vi "WS1050 VPI CP Sweep Cmd.vi"(8 "error in (no error)":errorcluster, 11 "x":dbl=23.0) -> (0 "error out":errorcluster, 2 "Bi_Voltage Out":string[](array[string]), 3 "Bi_Cmd Out":string[](array[string]), 4 "CP Sweep Cmd":string[](array[string]), 5 "Voltage(V)":string[](array[string]))   [LabVIEW 2012]
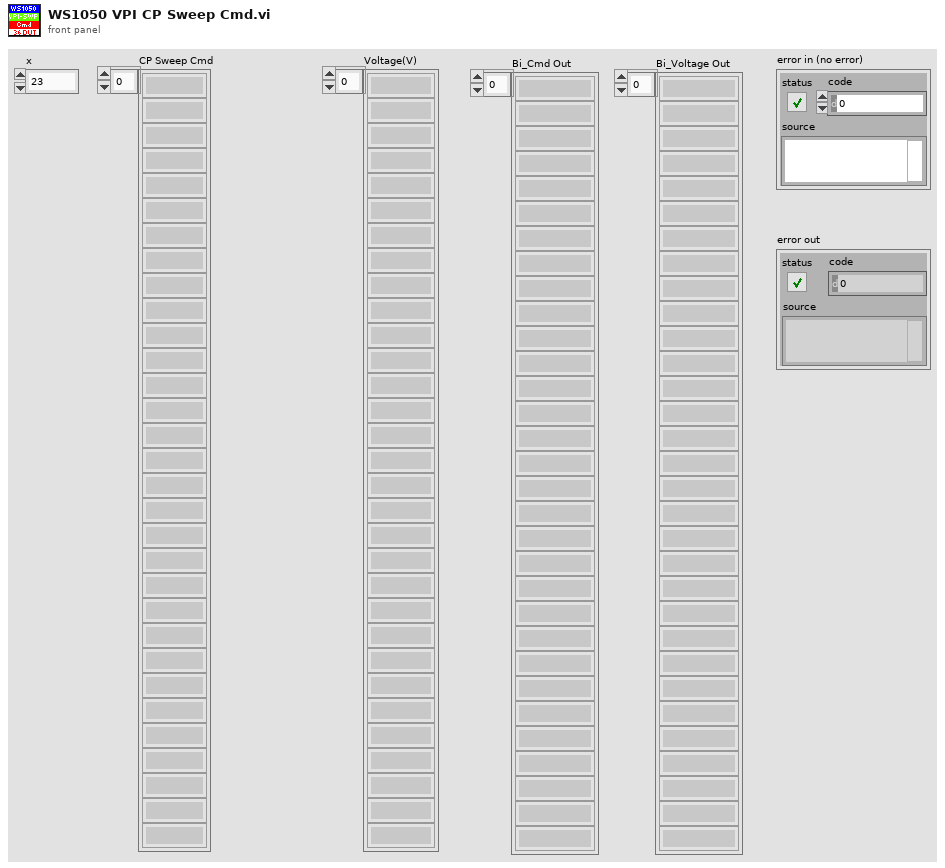
[diagram p1: front panel]
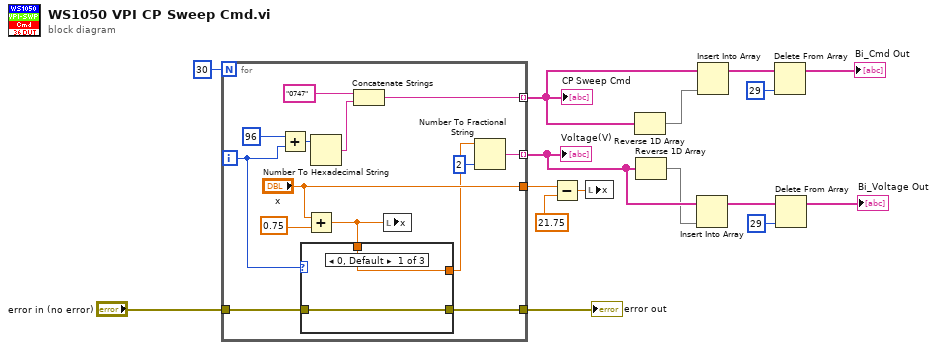
[diagram p0: block diagram]
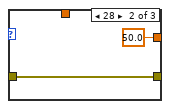
[diagram p2: hidden frame]
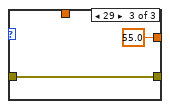
[diagram p3: hidden frame]
diagram:
  n1 = for {
    N: 30 -> [_]
    tunnel: [w26] -> w12 mode=indexing
    tunnel: ["x"] -> w15
    tunnel: [w20] -> w10 mode=indexing
    tunnel: "error in (no error)" -> [w18]
    tunnel: [w17] -> w1
    i -> [w24]
    n2 = Add(x=96, y=w24) -> (x+y=w29:i32)
    n3 = Add(x="x", y=0.75) -> (x+y=w23:dbl)
    n4 = case shown="0, Default" w24 {
      tunnel: [w32 50.0 55.0] -> w19
      tunnel: w23 -> [w32 _ _]
      tunnel: w18 -> [w31 w33 w35]
      tunnel: [w31 w33 w35] -> w17
      frame 0, Default {
      }
      frame 28 {
      }
      frame 29 {
      }
    }
    n5 = Number To Hexadecimal String(2:w29) -> (0:w27:string)  [unwired: 1 in]
    n6 = Concatenate Strings("0747", w27) -> (w26:string)
    n7 = local write "x"(w23) -> ()
    n8 = Number To Fractional String(number=w19, precision (6)=i16 2) -> (F-format string=w20:string)  [unwired: 2 in]
  }
  "CP Sweep Cmd" <- w12
  "Voltage(V)" <- w10
  "error out" <- w1
  n9 = Subtract(x=w15, y=21.75) -> (x-y=w13:dbl)
  n10 = local write "x"(w13) -> ()
  n11 = Reverse 1D Array(array=w12) -> (reversed array=w11:string[])
  n12 = Reverse 1D Array(array=w10) -> (reversed array=w9:string[])
  n13 = Insert Into Array(array=w10, new element=w9) -> (w4:string[])  [unwired: 1 in]
  n14 = Insert Into Array(array=w12, new element=w11) -> (w8:string[])  [unwired: 1 in]
  n15 = Delete From Array(array=w8, index=29 ("length")) -> (array with subset deleted=→"Bi_Cmd Out":string[])  [unwired: 1 in, 1 out]
  n16 = Delete From Array(array=w4, index=29 ("length")) -> (array with subset deleted=→"Bi_Voltage Out":string[])  [unwired: 1 in, 1 out]
